vi "HexFile@20260210.vi"(5 "Offset":cluster{"Angle":sgl, "AngEle":sgl, "RCS":sgl}[](array[cluster]), 6 "Data Log Path":path=path "D:/EOL3 Datas", 7 "SN":string="123", 8 "error in (no error)":errorcluster, 9 "Boolean":bool=TRUE, 10 "RFPayloads":u8[](array[numeric]) format="%.0x", 11 "calibration_parameters":T1[](array[typedef])=[{"re"=1.0, "im"=0.0}, {"re"=-0.96036863, "im"=0.2425586}, {"re"=0.9626107, "im"=-0.2713669}, {"re"=-0.58503306, "im"=0.7473227}, {"re"=1.0340631, "im"=-0.051051468}, {"re"=-0.9827397, "im"=0.29056582}, {"re"=0.9798006, "im"=-0.31922665}, {"re"=-0.5774226, "im"=0.79138196}, {"re"=0.83439076, "im"=0.47953746}, {"re"=-0.9034144, "im"=-0.2641089}, {"re"=0.9161487, "im"=0.24367115}, {"re"=-0.8432455, "im"=0.32213277}, {"re"=0.39170918, "im"=0.81630135}, {"re"=-0.566318, "im"=-0.6832286}, {"re"=0.58235455, "im"=0.6756262}, {"re"=-0.82617307, "im"=-0.19347626}]) -> (0 "error out":errorcluster, 3 "hex file path":path=path "D:/RadarTest/hex file/2026-02-10/[2026-02-10][17-42-55][123][CalHex].hex")   [LabVIEW 2024]
uses:
  Controls/Calc Para_float.ctl
panel:
  in  "re_imagePath":path=path "C:/Users/Radar/Desktop/EOL3/real-imag.csv"
  in  "Offset Path":path=path "C:/Users/Radar/Desktop/EOL3/Angle-Elv-RCS更新2.csv"
  in  "RFPath":path=path "C:/Users/Radar/Desktop/EOL3/RFData_New.csv"
  out "calibration_parameters_radar":i32[](array[numeric])=[32767, 0, 0, 0, 0, 0, 0, 0, 0, 0, 0, 0, 0, 0, 0, 0, 0, 0, 0, 0, 0, 0, 0, 0, 0, 0, 0, 0, 0, 0, 0, 0, 0, 0, -22022, 17412, 0, 0, 0, 0, 0, 0, 0, 0, 0, 0, 0, 0, 0, 0, 0, 0, 0, 0, 0, 0, 0, 0, 0, 0, 0, 0, 0, 0, 0, 0, 0, 0, -6428, 23081, 0, 0, 0, 0, 0, 0, 0, 0, 0, 0, 0, 0, 0, 0, 0, 0, 0, 0, 0, 0, 0, 0, 0, 0, 0, 0, 0, 0, 0, 0, 0, 0, 22438, 14859, 0, 0, 0, 0, 0, 0, 0, 0, 0, 0, 0, 0, 0, 0, 0, 0, 0, 0, 0, 0, 0, 0, 0, 0, 0, 0, 0, 0, 0, 0, 0, 0, 7094, 31223, 0, 0, 0, 0, 0, 0, 0, 0, 0, 0, 0, 0, 0, 0, 0, 0, 0, 0, 0, 0, 0, 0, 0, 0, 0, 0, 0, 0, 0, 0, 0, 0, -21658, -17350, 0, 0, 0, 0, 0, 0, 0, 0, 0, 0, 0, 0, 0, 0, 0, 0, 0, 0, 0, 0, 0, 0, 0, 0, 0, 0, 0, 0, 0, 0, 0, 0, -23661, -1107, 0, 0, 0, 0, 0, 0, 0, 0, 0, 0, 0, 0, 0, 0, 0, 0, 0, 0, 0, 0, 0, 0, 0, 0, 0, 0, 0, 0, 0, 0, 0, 0, -9377, 24883, 0, 0, 0, 0, 0, 0, 0, 0, 0, 0, 0, 0, 0, 0, 0, 0, 0, 0, 0, 0, 0, 0, 0, 0, 0, 0, 0, 0, 0, 0, 0, 0, -25469, 7041, 0, 0, 0, 0, 0, 0, 0, 0, 0, 0, 0, 0, 0, 0, 0, 0, 0, 0, 0, 0, 0, 0, 0, 0, 0, 0, 0, 0, 0, 0, 0, 0, 13549, -18588, 0, 0, 0, 0, 0, 0, 0, 0, 0, 0, 0, 0, 0, 0, 0, 0, 0, 0, 0, 0, 0, 0, 0, 0, 0, 0, 0, 0, 0, 0, 0, 0, -72, -19604, 0, 0, 0, 0, 0, 0, 0, 0, 0, 0, 0, 0, 0, 0, 0, 0, 0, 0, 0, 0, 0, 0, 0, 0, 0, 0, 0, 0, 0, 0, 0, 0, -20977, -6763, 0, 0, 0, 0, 0, 0, 0, 0, 0, 0, 0, 0, 0, 0, 0, 0, 0, 0, 0, 0, 0, 0, 0, 0, 0, 0, 0, 0, 0, 0, 0, 0, 18146, 23811, 0, 0, 0, 0, 0, 0, 0, 0, 0, 0, 0, 0, 0, 0, 0, 0, 0, 0, 0, 0, 0, 0, 0, 0, 0, 0, 0, 0, 0, 0, 0, 0, -25253, -6402, 0, 0, 0, 0, 0, 0, 0, 0, 0, 0, 0, 0, 0, 0, 0, 0, 0, 0, 0, 0, 0, 0, 0, 0, 0, 0, 0, 0, 0, 0, 0, 0, -20689, 8381, 0, 0, 0, 0, 0, 0, 0, 0, 0, 0, 0, 0, 0, 0, 0, 0, 0, 0, 0, 0, 0, 0, 0, 0, 0, 0, 0, 0, 0, 0, 0, 0, 1680, 24922]
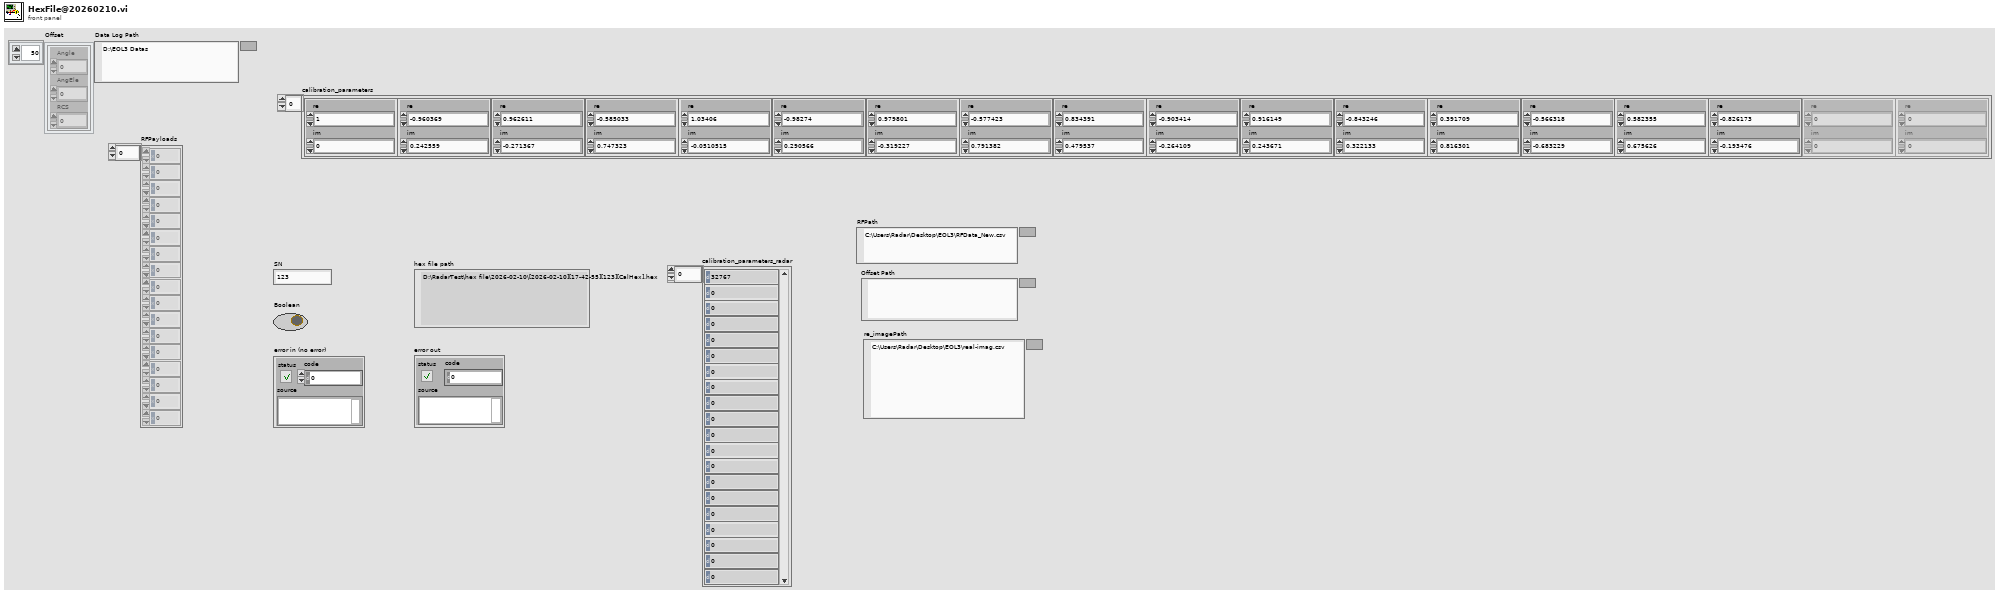
[diagram p1: front panel]
types:
  T1 = typedef "Calc Para_float.ctl" = cluster{"re":sgl, "im":sgl}
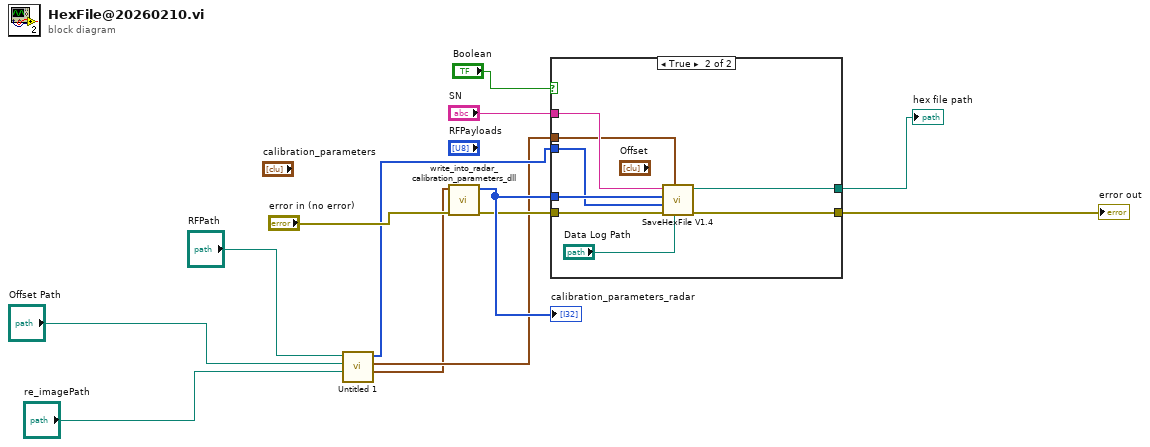
[diagram p0: block diagram]
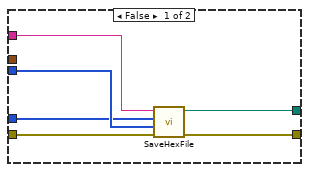
[diagram p2: hidden frame]
diagram:
  n1 = call "Untitled 1.vi"("re_imagePath"="re_imagePath", "Offset Path"="Offset Path", "RFPath"="RFPath") -> ("calibration_parameters"=w4:T1[], "Offset"=w5:cluster{"Angle":sgl, "AngEle":sgl, "RCS":sgl}[], "RF PayLoad"=w6:u8[])  [unwired: 6 in]
  n2 = call "write_into_radar_calibration_parameters_dll.vi"("error in (no error)"="error in (no error)", "calibration_parameters"=w4) -> ("error out"=w12:errorcluster, "calibration_parameters_radar"=w13:i32[])  [unwired: 7 in, 1 out]
  "calibration_parameters_radar" <- w13
  n3 = case shown="True" "Boolean" {
    tunnel: w13 -> [w14 w27]
    tunnel: w12 -> [w19 w26]
    tunnel: [w18 w25] -> w11
    tunnel: "SN" -> [w16 w24]
    tunnel: w6 -> [w15 w23]
    tunnel: [w17 w22] -> w8
    tunnel: w5 -> [_ w20]
    frame False {
      n4 = call "SaveHexFile.vi"("error IO"=w19, "RFPayloads"=w15, "calibration_parameters_radar"=w14, "SN"=w16) -> ("error out"=w18:errorcluster, "hex file path"=w17:path)  [unwired: 6 in]
    }
    frame True {
      n5 = call "SaveHexFile V1.4.vi"("Data Log Path"="Data Log Path", "Offset"=w20, "error IO"=w26, "RFPayloads"=w23, "calibration_parameters_radar"=w27, "SN"=w24) -> ("error out"=w25:errorcluster, "hex file path"=w22:path)  [unwired: 4 in]
    }
  }
  "error out" <- w11
  "hex file path" <- w8
